vi "m1m3_logEvent_HardpointActuatorWarning.vi"(8 "error in (no error)":errorcluster, 11 "logevent_HardpointActuatorWarning_Ctl":T1) -> (0 "error out":errorcluster, 2 "function return":i32, 3 "logevent_HardpointActuatorWarning_Ctl out":T1)   [LabVIEW 2016, in "SALLV_m1m3.lvlib"]
doc: "int m1m3_shm_logEvent_HardpointActuatorWarningLV(m1m3_logevent_HardpointActuatorWarningLV *logevent_HardpointActuatorWarning_Ctl );"
uses:
  SALLV_m1m3.lvlib
  DataTypes/logevent_HardpointActuatorWarning.ctl
  SALLV_m1m3.so
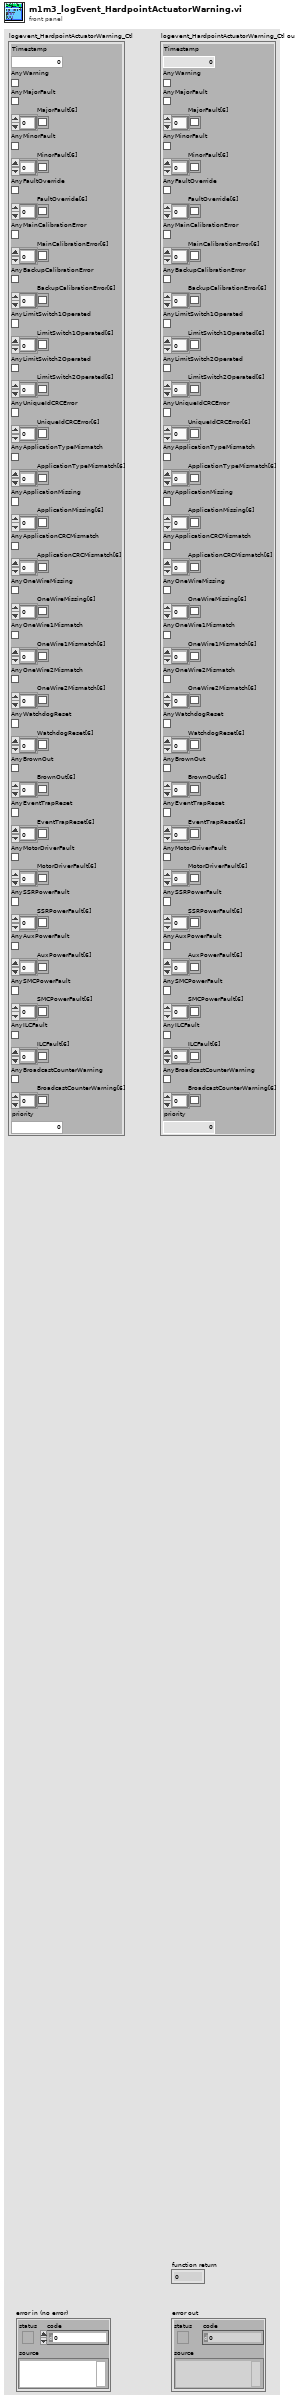
[diagram p1: front panel]
types:
  T1 = typedef "SALLV_m1m3.lvlib/logevent_HardpointActuatorWarning.ctl" = cluster{"Timestamp":dbl, "AnyWarning":bool, "AnyMajorFault":bool, "MajorFault[6]":bool[], "AnyMinorFault":bool, "MinorFault[6]":bool[], "AnyFaultOverride":bool, "FaultOverride[6]":bool[], "AnyMainCalibrationError":bool, "MainCalibrationError[6]":bool[], "AnyBackupCalibrationError":bool, "BackupCalibrationError[6]":bool[], "AnyLimitSwitch1Operated":bool, "LimitSwitch1Operated[6]":bool[], "AnyLimitSwitch2Operated":bool, "LimitSwitch2Operated[6]":bool[], "AnyUniqueIdCRCError":bool, "UniqueIdCRCError[6]":bool[], "AnyApplicationTypeMismatch":bool, "ApplicationTypeMismatch[6]":bool[], "AnyApplicationMissing":bool, "ApplicationMissing[6]":bool[], "AnyApplicationCRCMismatch":bool, "ApplicationCRCMismatch[6]":bool[], "AnyOneWireMissing":bool, "OneWireMissing[6]":bool[], "AnyOneWire1Mismatch":bool, "OneWire1Mismatch[6]":bool[], "AnyOneWire2Mismatch":bool, "OneWire2Mismatch[6]":bool[], "AnyWatchdogReset":bool, "WatchdogReset[6]":bool[], "AnyBrownOut":bool, "BrownOut[6]":bool[], "AnyEventTrapReset":bool, "EventTrapReset[6]":bool[], "AnyMotorDriverFault":bool, "MotorDriverFault[6]":bool[], "AnySSRPowerFault":bool, "SSRPowerFault[6]":bool[], "AnyAuxPowerFault":bool, "AuxPowerFault[6]":bool[], "AnySMCPowerFault":bool, "SMCPowerFault[6]":bool[], "AnyILCFault":bool, "ILCFault[6]":bool[], "AnyBroadcastCounterWarning":bool, "BroadcastCounterWarning[6]":bool[], "priority":i32}
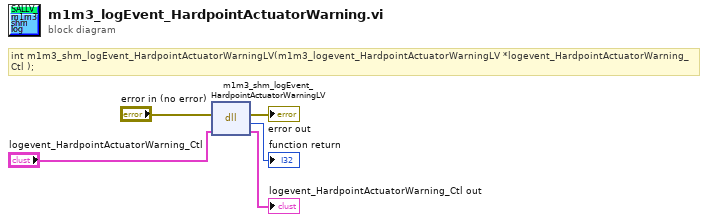
[diagram p0: block diagram]
diagram:
  # "int m1m3_shm_logEvent_HardpointActuatorWarningLV(m1m3_logevent_HardpointActuatorWarningLV *logevent_HardpointActuatorWarning_Ctl );"
  n1 = dll-call lib="opt/CODE/SALLV_m1m3/SALLV_m1m3.*" fn="m1m3_shm_logEvent_HardpointActuatorWarningLV"(error in="error in (no error)", "logevent_HardpointActuatorWarning_Ctl"="logevent_HardpointActuatorWarning_Ctl") -> (error out=→"error out":errorcluster, →"function return":i32, "logevent_HardpointActuatorWarning_Ctl"=→"logevent_HardpointActuatorWarning_Ctl out":T1)  [unwired: 2 in, 1 out]
